vi "FeedbackNode.vi"() -> ()   [LabVIEW 2021]
panel:
  out "Factorial2":i32
  out "Factorial":i32
  in  "Numeric":i32
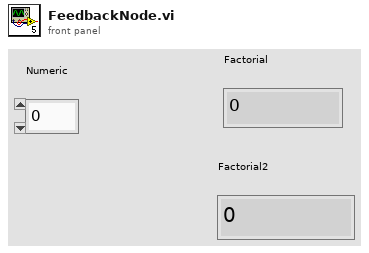
[diagram p1: front panel]
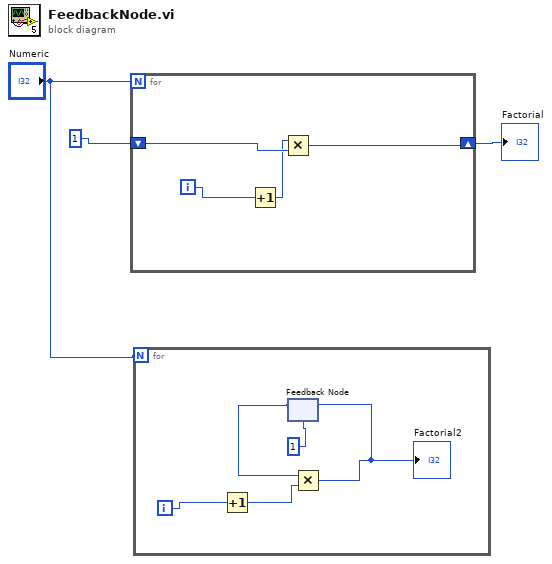
[diagram p0: block diagram]
diagram:
  n1 = for {
    N: "Numeric" -> [_]
    shift-right: [w4] -> w2
    shift-left: 1 -> [w6]
    i -> [w7]
    n2 = Increment(x=w7) -> (x+1=w5:i32)
    n3 = Multiply(x=w5, y=w6) -> (x*y=w4:i32)
  }
  "Factorial" <- w2
  n4 = for {
    N: "Numeric" -> [_]
    i -> [w12]
    n5 = Increment(x=w12) -> (x+1=w11:i32)
    n6 = feedback #1(1) -> (w9:i32)
    n7 = Multiply(x=w9, y=w11) -> (x*y=w10:i32)
    "Factorial2" <- w10
    n8 = feedback-in #1(w10) -> ()
  }
